vi "HMI Global to Cluster.vi"() -> (2 "HMI Cluster Out":T2)   [LabVIEW 2019]
uses:
  Globals and Definitions/HMI Typedef.ctl
  Globals and Definitions/RT Globals RD v1.0.vi
  Globals and Definitions/Initialization Globals.vi
panel:
  in  "Packet 20 Decoded Data Cluster 2":T1
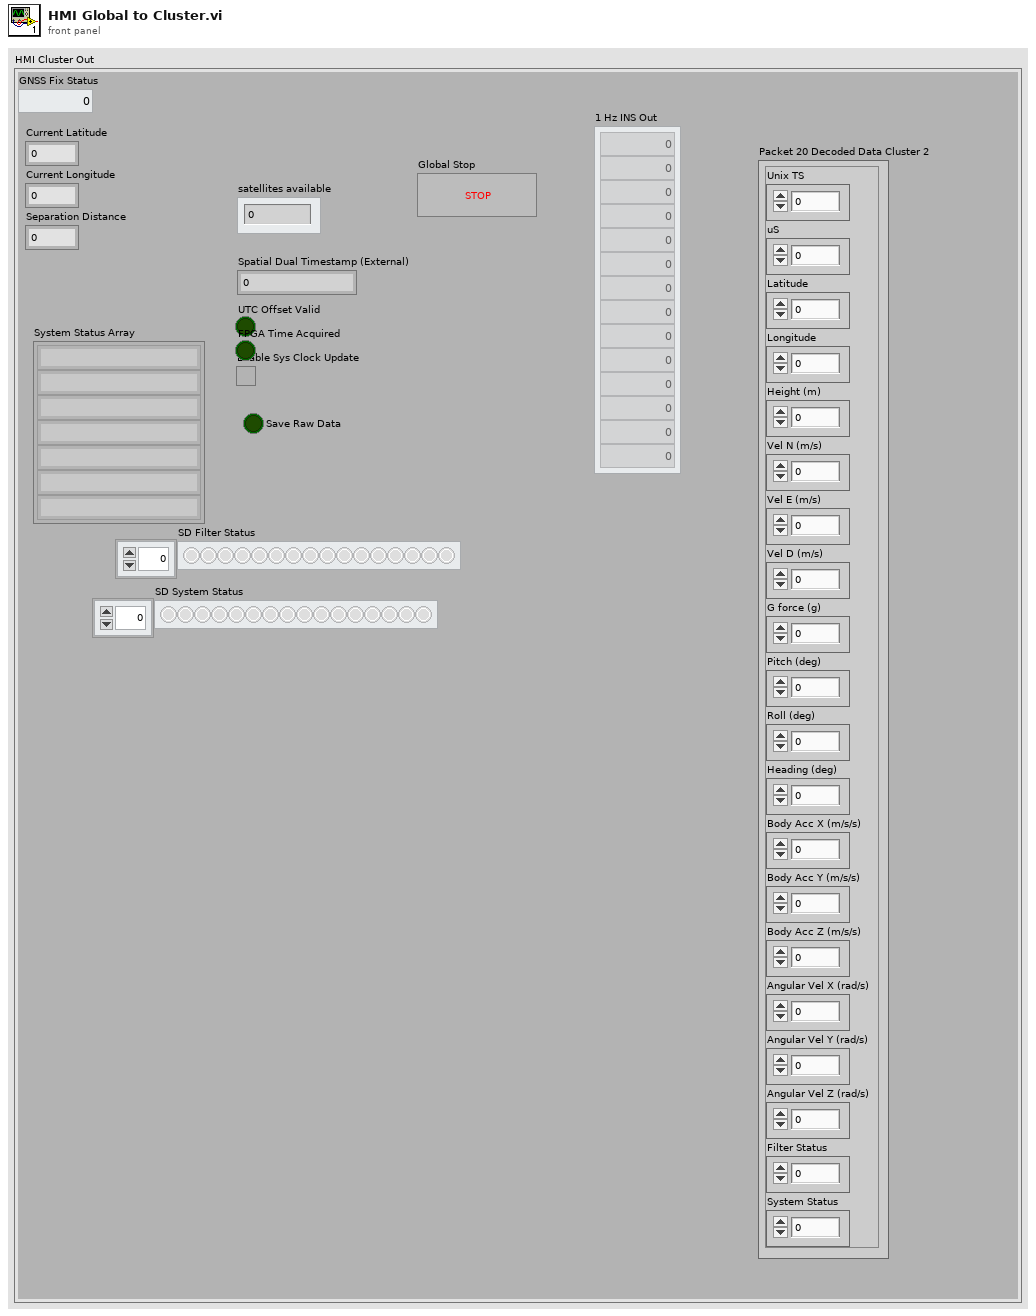
[diagram p1: front panel]
types:
  T1 = cluster{"Unix TS":u32, "uS":u32, "Latitude":dbl, "Longitude":dbl, "Height (m)":dbl, "Vel N (m/s)":sgl, "Vel E (m/s)":sgl, "Vel D (m/s)":sgl, "G force (g)":sgl, "Pitch (deg)":sgl, "Roll (deg)":sgl, "Heading (deg)":sgl, "Body Acc X (m/s/s)":sgl, "Body Acc Y (m/s/s)":sgl, "Body Acc Z (m/s/s)":sgl, "Angular Vel X (rad/s)":sgl, "Angular Vel Y (rad/s)":sgl, "Angular Vel Z (rad/s)":sgl, "Filter Status":u16, "System Status":u16}
  T2 = typedef "HMI Typedef.ctl" = cluster{"Current Latitude":dbl, "Current Longitude":dbl, "Separation Distance":dbl, "Global Stop":bool, "UTC Offset Valid":bool, "1 Hz INS Out":dbl[], "GNSS Fix Status":u32, "satellites available":u8, "System Status Array":string[], "Enable Sys Clock Update":bool, "Spatial Dual Timestamp (External)":u64, "SD Filter Status":bool[], "SD System Status":bool[], "FPGA Time Acquired":bool, "Save Raw Data":bool}
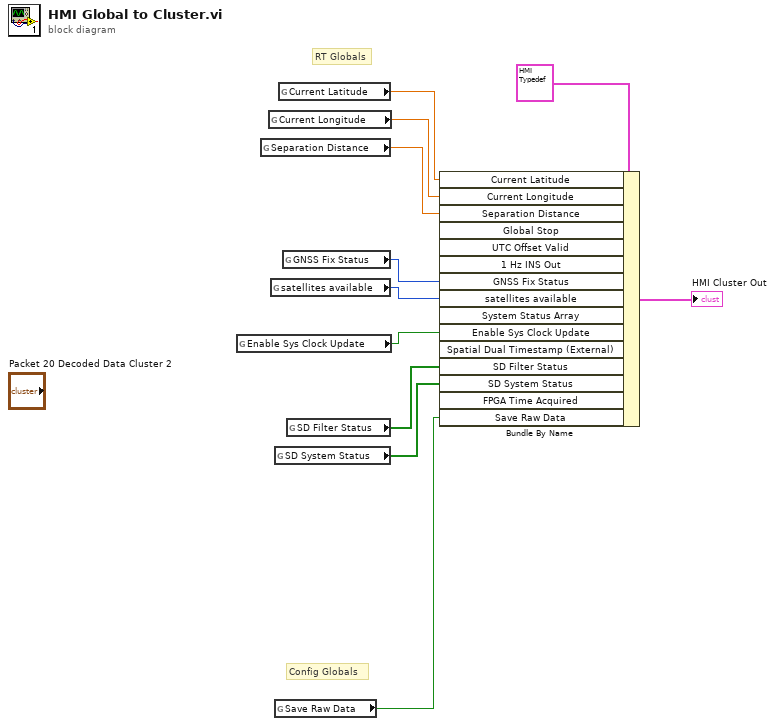
[diagram p0: block diagram]
diagram:
  # "Config Globals"
  # "RT Globals"
  n1 = global read "RT Globals RD v1.0.vi" "Enable Sys Clock Update"() -> (w6:bool)
  n2 = global read "RT Globals RD v1.0.vi" "Separation Distance"() -> (w9:dbl)
  n3 = global read "RT Globals RD v1.0.vi" "Current Longitude"() -> (w10:dbl)
  n4 = global read "RT Globals RD v1.0.vi" "satellites available"() -> (w7:u8)
  n5 = global read "RT Globals RD v1.0.vi" "SD System Status"() -> (w4:bool[])
  n6 = global read "Initialization Globals.vi" "Save Raw Data"() -> (w1:bool)
  n7 = global read "RT Globals RD v1.0.vi" "Current Latitude"() -> (w11:dbl)
  n8 = global read "RT Globals RD v1.0.vi" "GNSS Fix Status"() -> (w8:u32)
  n9 = global read "RT Globals RD v1.0.vi" "SD Filter Status"() -> (w5:bool[])
  n10 = Bundle By Name(cluster=T2 {"Current Latitude"=0.0, "Current Longitude"=0.0, "Separation Distance"=0.0, "Global Stop"=FALSE, "UTC Offset Valid"=FALSE, "1 Hz INS Out"=[], "GNSS Fix Status"=0, "satellites available"=0, "System Status Array"=[], "Enable Sys Clock Update"=FALSE, "Spatial Dual Timestamp (External)"=0, "SD Filter Status"=[], "SD System Status"=[], "FPGA Time Acquired"=FALSE, "Save Raw Data"=FALSE} ("HMI Data Cluster"), "Current Latitude"=w11, "Current Longitude"=w10, "Separation Distance"=w9, "GNSS Fix Status"=w8, "satellites available"=w7, "Enable Sys Clock Update"=w6, "SD Filter Status"=w5, "SD System Status"=w4, "Save Raw Data"=w1) -> (→"HMI Cluster Out":T2)  [unwired: 6 in]
